vi "AutoJump.vi"(6 "Current Index":i32, 10 "Goto":i32, 11 "Type":i32) -> (1 "Done?":bool, 4 "New Index":i32)   [LabVIEW 2014]
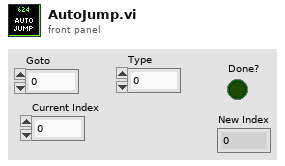
[diagram p1: front panel]
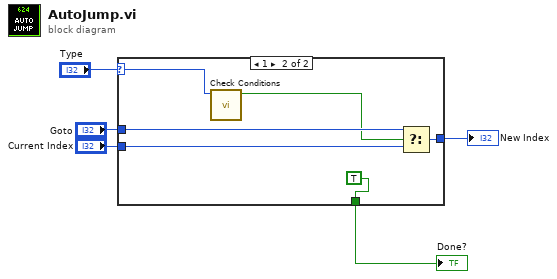
[diagram p0: block diagram]
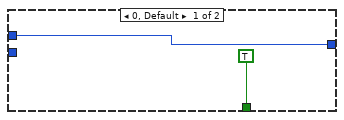
[diagram p2: hidden frame]
diagram:
  n1 = case shown="1" "Type" {
    selector: "Type" -> [_ w9]
    tunnel: [w7 w11] -> w4
    tunnel: "Goto" -> [w7 w12]
    tunnel: [TRUE TRUE] -> w2
    tunnel: "Current Index" -> [_ w13]
    frame 0, Default {
    }
    frame 1 {
      n2 = call "Check Conditions.vi"("Condition"=w9) -> ("Done?"=w8:bool)  [unwired: 10 in]
      n3 = Select(t=w12, s=w8, f=w13) -> (s? t:f=w11:i32)
    }
  }
  "Done?" <- w2
  "New Index" <- w4
